vi "Contents Summary Text.vi"(11 "Message":refnum<class "ObserverRegistryCommand.lvclass">) -> (2 "Contents Summary Text":string, 3 "Message":refnum<class "ObserverRegistryCommand.lvclass">)   [LabVIEW 2011, in "Messenging.lvlib" / "ObserverRegistryCommand.lvclass"]
uses:
  ObserverRegistryCommand.lvclass
  Interprocess Messenger/Send/Send.lvclass
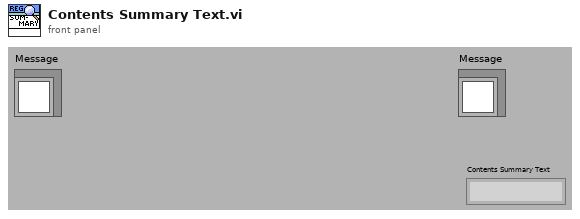
[diagram p1: front panel]
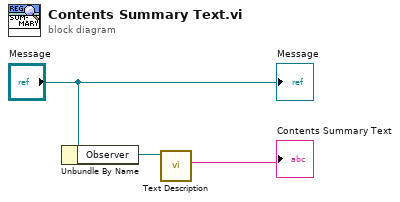
[diagram p0: block diagram]
diagram:
  n1 = Unbundle By Name("Message") -> ("Observer"=w2:refnum<class "Send.lvclass">)
  n2 = call-dynamic "Text Description.vi"("Send in"=w2) -> ("Description"=→"Contents Summary Text":string)  [unwired: 10 out]
  "Message" <- "Message"
